vi "Read Offline Data.vi"(8 "Error In":errorcluster) -> (0 "Error Out":errorcluster)   [LabVIEW 2014, in "Aquisicao de Dados.lvlib"]
uses:
  Aquisicao de Dados.lvlib
  <vilib>/express/express analysis/Spectral/Block/exnSpectralBlock spectral measurements peak poly.vi
  <vilib>/express/express analysis/Spectral/Block/exnSpectralBlock spectral measurements peak WFM.vi
  <vilib>/express/express analysis/Spectral/XNode/ExpressSpectralMeasurementsBlockNode.xnode
panel:
  out "x-y":dbl
  out "F5 (Hz)":dbl
  out "A5 (V)":dbl
  out "F4 (Hz)":dbl
  out "A4 (V)":dbl
  out "F3 (Hz)":dbl
  out "A3 (V)":dbl
  out "F2 (Hz)":dbl
  out "A2 (V)":dbl
  out "F1 (Hz)":dbl
  out "A1 (V)":dbl
  out "Period dt":dbl
  out "FFT Overview":cluster{"f0":dbl, "df":dbl, "magnitude":dbl[]}(graph)
  out "Y min":dbl format="%0.2f"
  out "Y max":dbl format="%0.2f"
  out "Output Audio":waveform(dbl)(graph)
  out "Measured Fs":dbl
  out "Canal 1":waveform(dbl)(graph)
  out "Canal 0":waveform(dbl)(graph)
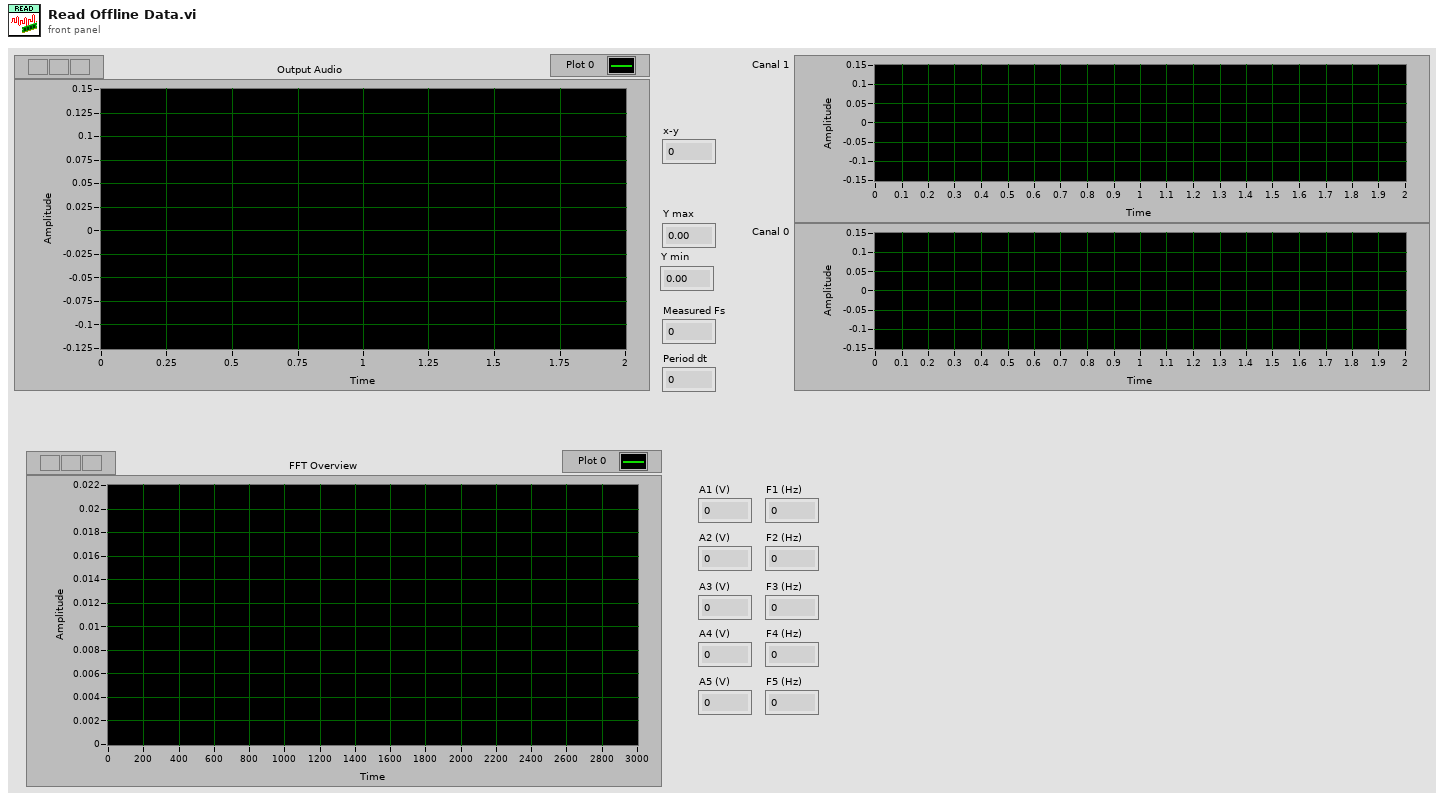
[diagram p1: front panel]
types:
  T1 = enum32{".WAV File", "LTSpice Simulation", "Microphone", "MultiSim Simulation", "Serial Port"}
  T2 = typedef "Aquisicao de Dados.lvlib/_ACC_DATA_ Config DAta State.ctl" = cluster{"_RAW_ Traces":cluster{"Trace Name":string, "Trace Type":string, "Trace Raw Data":dbl[], "Trace Waveform":waveform(dbl)}[], "_WAV_ Traces":waveform(dbl)[], "_MIC_ Config":cluster{"task ID":T3, "Data Chunk Size":i32, "Num Channels":i32, "Resolution":i32, "Sampling Frequency":dbl, "device ID":u32, "Num Chunks":i32}, "_LVM_ Traces":cluster{"Trace Name":string, "Trace Type":string, "Trace Raw Data":dbl[], "Trace Waveform":waveform(dbl)}[]}
  T3 = typedef "Sound Input Task ID.ctl" = u32
  T4 = typedef "LVCursorListTypeDef.ctl" = cluster{"Name":string, "Color":u32, "Style":u8, "Point Style":u8, "Name Visible":bool, "Allow Drag":bool, "Cursor Mode":u32, "Plot":i32, "Index":i32, "Position":cluster{"X":dbl, "Y":dbl}, "X Scale":u32, "Y Scale":u32, "Watch Plots":i32[], "Watch All Plots":bool, "Plot Area":i32, "Label Offset":cluster{"X":dbl, "Y":dbl}}[]
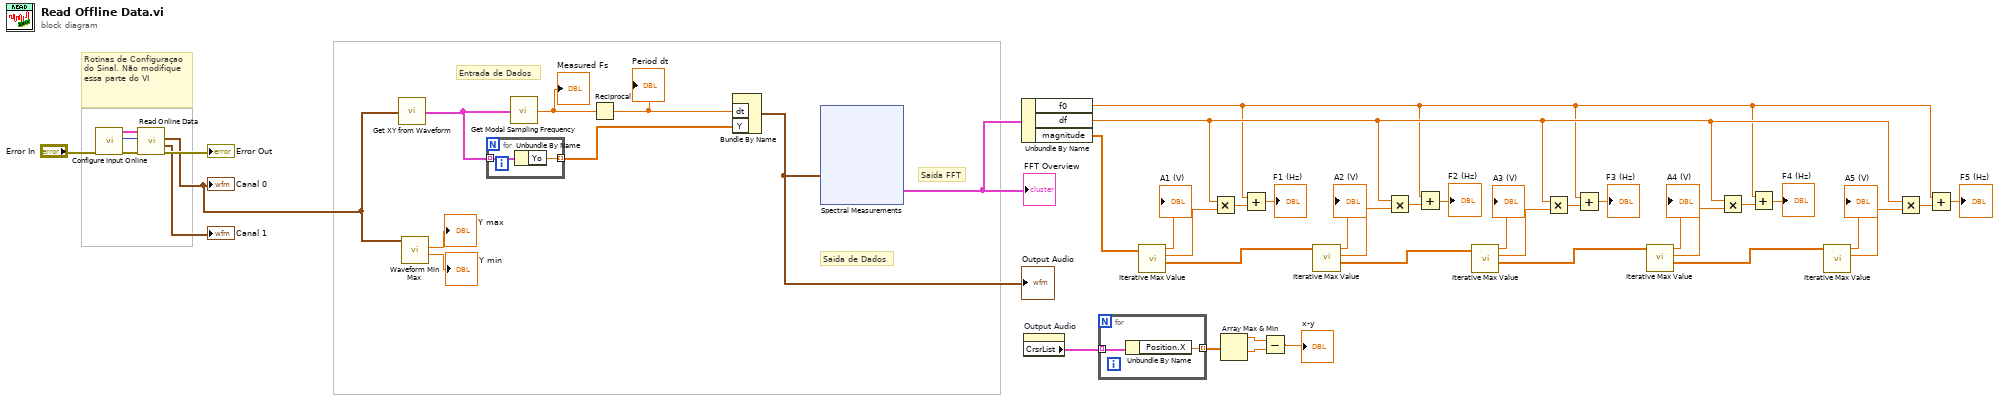
[diagram p0: block diagram]
diagram:
  # "Saída FFT"
  # "Saida de Dados"
  # "Entrada de Dados"
  # "Rotinas de Configuraçao do Sinal. Não modifique essa parte do VI"
  n1 = call "Configure Input Online.vi"("Error In"="Error In") -> ("Error Out"=w47:errorcluster, "Metodo de Entrada"=w45:T1, "Config Out"=w43:T2)  [unwired: 8 in]
  n2 = call "Read Online Data.vi"("Error In"=w47, "Metodo de Entrada"=w45, "Config Out"=w43) -> ("Error Out"=→"Error Out":errorcluster, "Channel 1"=→"Canal 1":waveform(dbl), "Channel 0"=w34:waveform(dbl))  [unwired: 6 in]
  "Canal 0" <- w34
  n3 = call "Get XY from Waveform.vi"("Waveform In"=w34) -> ("XY Array Out"=w39:cluster{"Yo":dbl, "Xo":timestamp}[])
  n4 = call <vilib>:"Waveform Min Max.vi"("waveform in"=w34) -> ("Y min"=→"Y min":dbl, "Y max"=→"Y max":dbl)  [unwired: 5 in, 4 out]
  n5 = for {
    tunnel: w39 -> [w49] mode=indexing
    tunnel: [w48] -> w42 mode=indexing
    n6 = Unbundle By Name(w49) -> ("Yo"=w48:dbl)
  }
  n7 = call "Get Modal Sampling Frequency.vi"("XY Data In"=w39) -> ("Measured Fs"=w40:dbl)
  "Measured Fs" <- w40
  n8 = Reciprocal(x=w40) -> (1/x=w41:dbl)
  "Period dt" <- w41
  n9 = Bundle By Name("dt"=w41, "Y"=w42) -> (w35:waveform(dbl))  [unwired: 1 in]
  "Output Audio" <- w35
  n10 = xnode "Spectral Measurements"("Signals"=w35) -> ("FFT - (Peak)"=w33:cluster{"f0":dbl, "df":dbl, "magnitude":dbl[]})  [unwired: 1 in, 2 out]
  "FFT Overview" <- w33
  n11 = Unbundle By Name(w33) -> ("f0"=w7:dbl, "df"=w8:dbl, "magnitude"=w32:dbl[])
  n12 = property on="Output Audio" class="WFGraph (strict)"() -> ("CrsrList"=w5:T4)  [unwired: 2 in, 2 out]
  n13 = for {
    tunnel: w5 -> [w51] mode=indexing
    tunnel: [w50] -> w4 mode=indexing
    n14 = Unbundle By Name(w51) -> ("Position.X"=w50:dbl)
  }
  n15 = call "Iterative Max Value.vi"("Array in"=w32) -> ("Array out"=w23:dbl[], "Max index"=w30:dbl, "Max value"=→"A1 (V)":dbl)  [unwired: 8 in]
  n16 = Multiply(x=w8, y=w30) -> (x*y=w28:dbl)
  n17 = Array Max & Min(array=w4) -> (max value=w3:dbl, min value=w2:dbl)  [unwired: 2 out]
  n18 = Add(x=w7, y=w28) -> (x+y=→"F1 (Hz)":dbl)
  n19 = Subtract(x=w3, y=w2) -> (x-y=→"x-y":dbl)
  n20 = call "Iterative Max Value.vi"("Array in"=w23) -> ("Array out"=w13:dbl[], "Max index"=w26:dbl, "Max value"=→"A2 (V)":dbl)  [unwired: 8 in]
  n21 = Multiply(x=w8, y=w26) -> (x*y=w24:dbl)
  n22 = Add(x=w7, y=w24) -> (x+y=→"F2 (Hz)":dbl)
  n23 = call "Iterative Max Value.vi"("Array in"=w13) -> ("Array out"=w14:dbl[], "Max index"=w21:dbl, "Max value"=→"A3 (V)":dbl)  [unwired: 8 in]
  n24 = Multiply(x=w8, y=w21) -> (x*y=w19:dbl)
  n25 = Add(x=w7, y=w19) -> (x+y=→"F3 (Hz)":dbl)
  n26 = call "Iterative Max Value.vi"("Array in"=w14) -> ("Array out"=w6:dbl[], "Max index"=w17:dbl, "Max value"=→"A4 (V)":dbl)  [unwired: 8 in]
  n27 = Multiply(x=w8, y=w17) -> (x*y=w15:dbl)
  n28 = Add(x=w7, y=w15) -> (x+y=→"F4 (Hz)":dbl)
  n29 = call "Iterative Max Value.vi"("Array in"=w6) -> ("Max index"=w11:dbl, "Max value"=→"A5 (V)":dbl)  [unwired: 8 in, 1 out]
  n30 = Multiply(x=w8, y=w11) -> (x*y=w9:dbl)
  n31 = Add(x=w7, y=w9) -> (x+y=→"F5 (Hz)":dbl)
